vi "Stop Core.vi"(10 "final error code":i32, 11 "Mag Lab Root in":refnum<class "Mag Lab Root.lvclass">) -> (3 "Mag Lab Root out":refnum<class "Mag Lab Root.lvclass">)   [LabVIEW 2015, in "Mag Lab Root.lvclass"]
doc: "(<B>Filename</B>: Actor Framework.lvlib:Actor.lvclass:Stop Core.vi)\n\nDefines what the actor does before it stops. Use the <B>final error code</B> input to determine whether the actor shut down in response to an error.\n\nBy default, this method does nothing. A descendant class may override it to define behavior, such as shutting down any processes the actor initiated in its override of the Actor Core method."
uses:
  Mag Lab Root.lvclass
  Mag Lab Root.lvclass/Mag Lab Root.ctl
  <vilib>/ActorFramework/Actor/Actor.lvclass
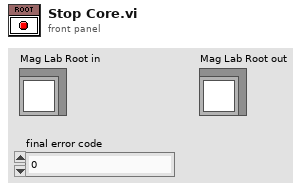
[diagram p1: front panel]
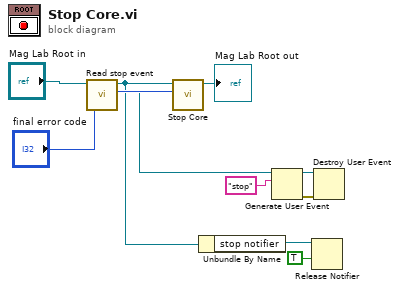
[diagram p0: block diagram]
diagram:
  n1 = call "Read stop event.vi"("Mag Lab Root in"="Mag Lab Root in") -> ("stop event"=w4:refnum<user-event>, "Mag Lab Root out"=w1:refnum<class "Mag Lab Root.lvclass">)  [unwired: 8 in, 1 out]
  n2 = call-parent "Stop Core.vi"("final error code"="final error code", "Actor in"=w1) -> ("Actor out"=→"Mag Lab Root out":refnum<class "Mag Lab Root.lvclass">)  [unwired: 9 in]
  n3 = Unbundle By Name(w1) -> ("stop notifier"=w3:refnum<notifier>)
  n4 = Generate User Event(user event=w4, event data cluster="stop" ("event data")) -> (user event out=w8:refnum<user-event>, error out=w7:errorcluster)  [unwired: 2 in]
  n5 = Release Notifier(notifier=w3, force destroy? (F)=TRUE) -> ()  [unwired: 1 in, 3 out]
  n6 = Destroy User Event(user event=w8, error in=w7) -> ()  [unwired: 1 out]
